vi "SaveAs.vi"(8 "error in":errorcluster, 11 "state in":T1) -> (0 "error out":errorcluster, 1 "canceled?":bool, 3 "state out":T1)   [LabVIEW 2014, in "CI Project Builder.lvlib"]
doc: "Calls the Save Dialog VI, and if a valid names is given calls the save function."
uses:
  CI Project Builder.lvlib
  Controls/StateCluster.ctl
  <vilib>/ni/Configuration Framework/Node/NodeRef.ctl
  <vilib>/ni/Configuration Framework/Node/NISE_CEF_Node.lvclass
  <vilib>/ni/Configuration Framework/Node/StandardEvents.ctl
  <vilib>/ni/Configuration Framework/Node/UserEventRef.ctl
  <vilib>/ni/Configuration Framework/Controls/EventCluster.ctl
  <vilib>/ni/Configuration Framework/Node/NodeChangeEvent.ctl
  <vilib>/ni/Configuration Framework/Node/CacheState.ctl
  <vilib>/ni/Configuration Framework/Node/RefreshUIEvent.ctl
  <vilib>/ni/Configuration Framework/Node/StopEvent.ctl
  <vilib>/ni/Configuration Framework/glyph manager/glyph manager.ctl
  <vilib>/picture/picture.llb/imagedata.ctl
  Classes/INI Serializer/INI Serializer.lvclass
  Classes/CI Serializer/CI Serializer.lvclass
  <vilib>/ni/Configuration Framework/NISE_CEF_TreeControl.lvlib
  <vilib>/ni/Configuration Framework/glyph manager/glyph manager.lvlib
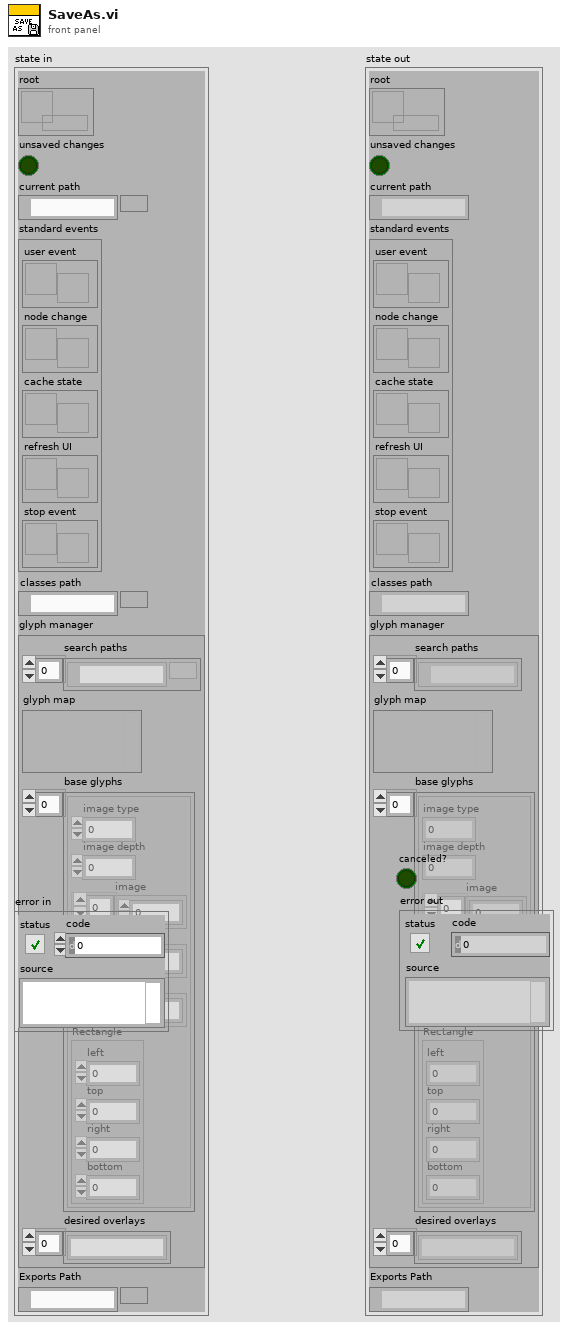
[diagram p1: front panel]
types:
  T1 = typedef "CI Project Builder.lvlib/StateCluster.ctl" = cluster{"root":T2, "unsaved changes":bool, "current path":path, "standard events":T3, "classes path":path, "glyph manager":T9, "Exports Path":path}
  T2 = typedef "NISE_CEF_Node.lvclass/NodeRef.ctl" = refnum<data-value>
  T3 = typedef "NISE_CEF_Node.lvclass/StandardEvents.ctl" = cluster{"user event":T4, "node change":T5, "cache state":T6, "refresh UI":T7, "stop event":T8}
  T4 = typedef "NISE_CEF_Node.lvclass/UserEventRef.ctl" = refnum<user-event>
  T5 = typedef "NISE_CEF_Node.lvclass/NodeChangeEvent.ctl" = refnum<user-event>
  T6 = typedef "NISE_CEF_Node.lvclass/CacheState.ctl" = refnum<user-event>
  T7 = typedef "NISE_CEF_Node.lvclass/RefreshUIEvent.ctl" = refnum<user-event>
  T8 = typedef "NISE_CEF_Node.lvclass/StopEvent.ctl" = refnum<user-event>
  T9 = typedef "glyph manager.lvlib/glyph manager.ctl" = cluster{"search paths":path[], "glyph map":variant, "base glyphs":T10[], "desired overlays":string[]}
  T10 = typedef "imagedata.ctl" = cluster{"image type":i32, "image depth":i32, "image":u8[], "mask":u8[], "colors":u32[], "Rectangle":cluster{"left":i16, "top":i16, "right":i16, "bottom":i16}}
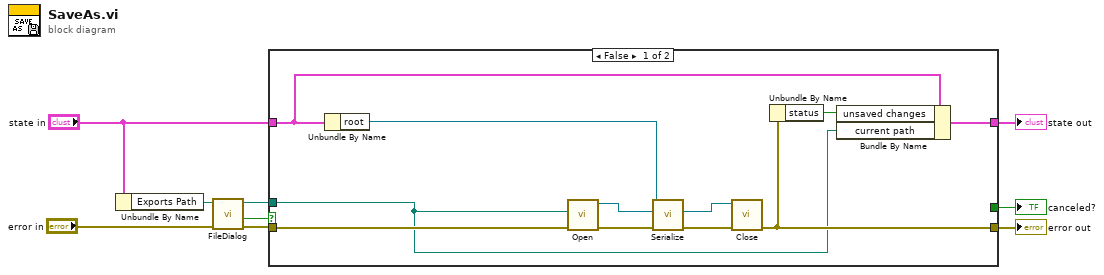
[diagram p0: block diagram]
diagram:
  n1 = Unbundle By Name("state in") -> ("Exports Path"=w1:path)
  n2 = call "FileDialog.vi"("error in"="error in", "start path"=w1) -> ("error out"=w6:errorcluster, "cancelled"=w4:bool, "selected path"=w5:path)  [unwired: 7 in]
  n3 = case shown="False" w4 {
    selector: w4 -> [_ w22]
    tunnel: "state in" -> [w20 w23]
    tunnel: w6 -> [w18 w21]
    tunnel: [w17 w21] -> w9
    tunnel: [w19 w23] -> w8
    tunnel: w5 -> [w15 _]
    tunnel: [_ w22] -> w3
    frame False {
      n4 = Unbundle By Name(w20) -> ("root"=w10:T2)
      n5 = call "Open.vi"("error in (no error)"=w18, "INI Path"=w15) -> ("error out"=w14:errorcluster, "INI Serializer out"=w13:refnum<class "INI Serializer.lvclass">)  [unwired: 8 in]
      n6 = call "Serialize.vi"("error in (no error)"=w14, "CI Serializer in"=w13, "Root Node"=w10) -> ("error out"=w11:errorcluster, "CI Serializer out"=w12:refnum<class "INI Serializer.lvclass">)  [unwired: 7 in]
      n7 = call "Close.vi"("error in (no error)"=w11, "INI Serializer in"=w12) -> ("error out"=w17:errorcluster)  [unwired: 9 in]
      n8 = Unbundle By Name(w17) -> ("status"=w16:bool)
      n9 = Bundle By Name(cluster=w20, "unsaved changes"=w16, "current path"=w15) -> (w19:T1)
    }
    frame True {
    }
  }
  "state out" <- w8
  "error out" <- w9
  "canceled?" <- w3
